vi "Joysticks In Range.vi"(8 "Range (.25)":dbl=0.25, 10 "y":dbl, 11 "x":dbl) -> (3 "x .and. y?":bool)   [LabVIEW 2015]
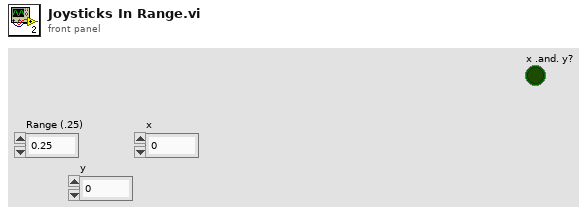
[diagram p1: front panel]
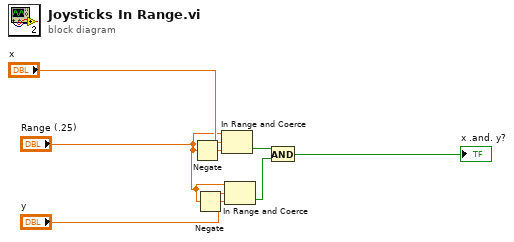
[diagram p0: block diagram]
diagram:
  n1 = Negate(x="Range (.25)") -> (-x=w8:dbl)
  n2 = Negate(x="Range (.25)") -> (-x=w5:dbl)
  n3 = In Range and Coerce(upper limit="Range (.25)", x="x", lower limit=w8) -> (In Range?=w7:bool)  [unwired: 1 out]
  n4 = In Range and Coerce(upper limit="Range (.25)", x="y", lower limit=w5) -> (In Range?=w2:bool)  [unwired: 1 out]
  n5 = And(x=w7, y=w2) -> (x .and. y?=→"x .and. y?":bool)
